vi "helper--Tag Editor.vi"() -> ()   [LabVIEW 2021]
doc: "set the control tags correctly for all of the button types in the directory\n\n<b>Code Developed By:</b>\nTechnology Service Corporation\n1983 S Liberty Drive\nBloomington, IN 47403\nPhone: 812 558-7100\nwww.tsc.com/atcs\n\nDeveloper:\nDaniel Coons"
panel:
  in  "write":bool
  out "Table Control":string[][](table)
  in  "Control":u16(ring) items=["elevated--rectangular--icon.ctl", "elevated--rounded--icon.ctl", "filled--rectangular--icon.ctl", "filled--rounded--icon.ctl", "nooutline--rectangular--icon.ctl", "nooutline--rounded--icon.ctl", "outline--rectangular--icon.ctl", "outline--rounded--icon.ctl", "tonal--rectangular--icon.ctl", "tonal--rounded--icon.ctl", "transparent--rectangular--icon.ctl", "transparent--rounded--icon.ctl", "FAB--icon--rounded.ctl", "nooutline--icon--rectangular--40x40.ctl", "filled--icon--mulitple--rectangular.ctl", "filled--text--rectangular.ctl", "filled--text--rounded.ctl", "nooutline--text--rectangular.ctl", "nooutline--text--rounded.ctl", "outline--text--rectangular.ctl", "outline--text--rounded.ctl", "tonal--text--rectangular.ctl", "tonal--text--rounded.ctl", "token--dark.ctl", "token--light.ctl"]
  in  "Tag Choice":string(combo)
  in  "Tag Value":string="button-type"
  out "error out":errorcluster
  # "legacy categories"
  # "control-level:\nN/A\nPrimary\nSecondary\nTertiary\nError\nPrimary Fixed\nSecondary Fixed\nTertiary Fixed"
  # "boolean-level:\nDefault\nN/A\nNo Change\nNo-Change\nNoChange\nNA"
  # "button-type:\nOutline\nNo-Outline\nTonal\nFilled\nTransparent\nFAB\nElevated"
  # "Control Types:\noutline--icon--rounded\noutline--text--rounded\nnooutline--icon--rounded\nnooutline--text--rounded\ntonal--icon--rounded\ntonal--text--rounded\nfilled--icon--rounded\nfilled--text--rounded"
  # "Control Types:\noutline--icon--rectangular\noutline--text--rectangular\nnooutline--icon--rectangular\nnooutline--text--rectangular\ntonal--icon--rectangular\ntonal--text--rectangular\nfilled--icon--rectangular\nfilled--text--rectangular"
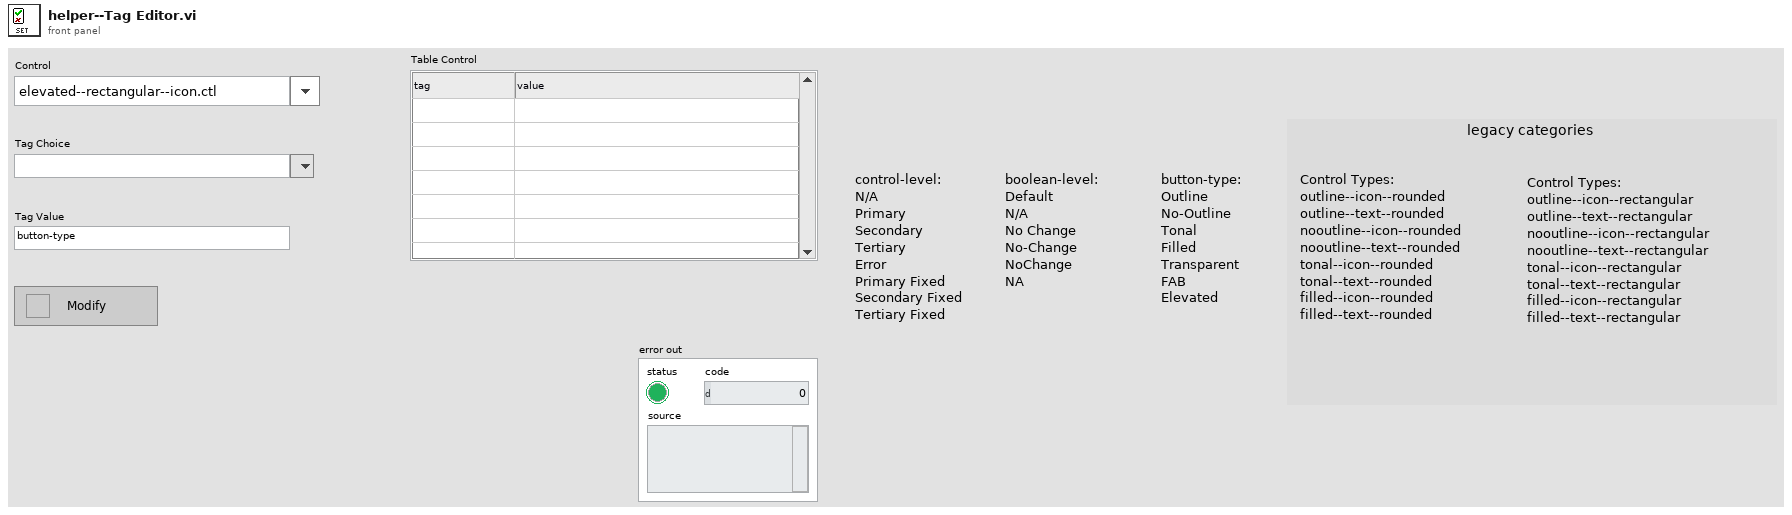
[diagram p1: front panel]
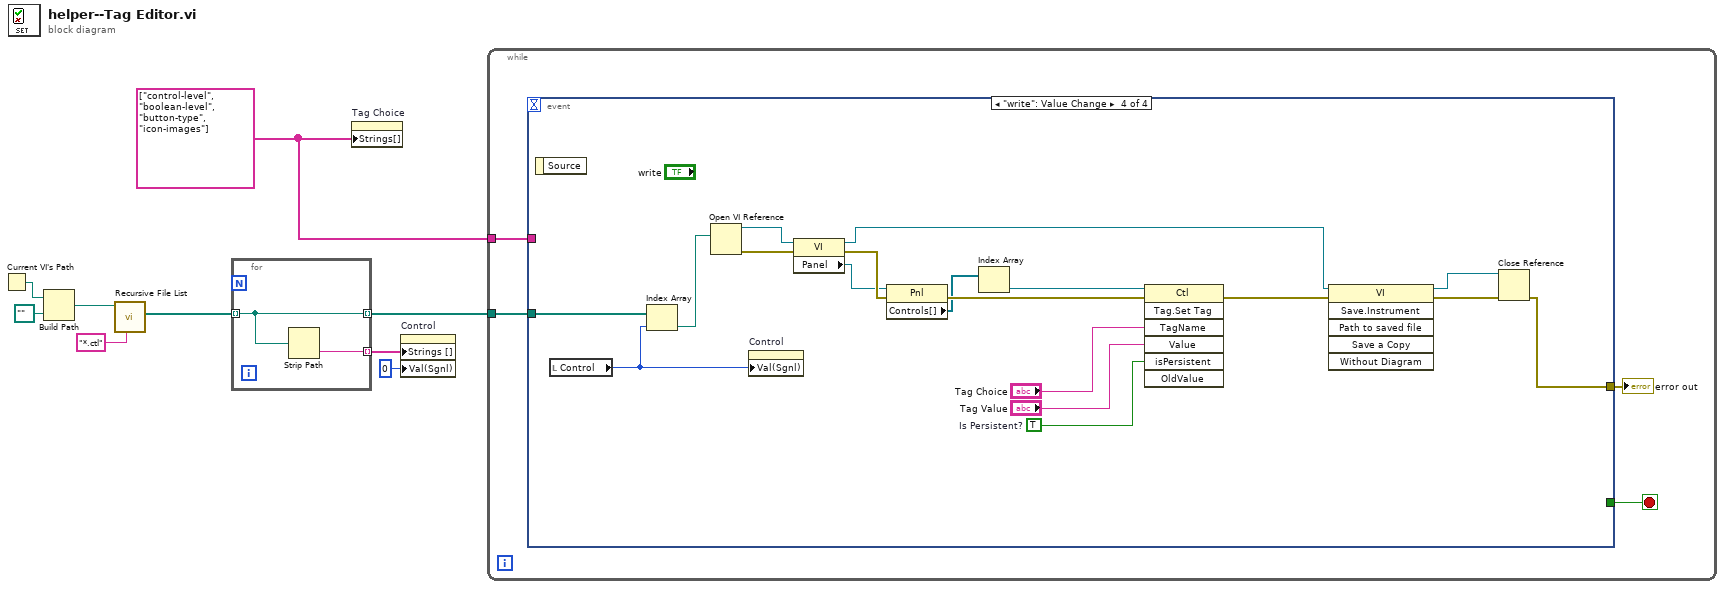
[diagram p0: block diagram]
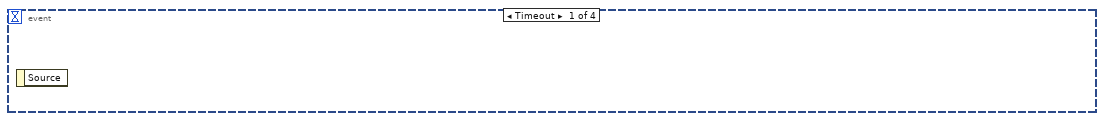
[diagram p2: hidden frame]
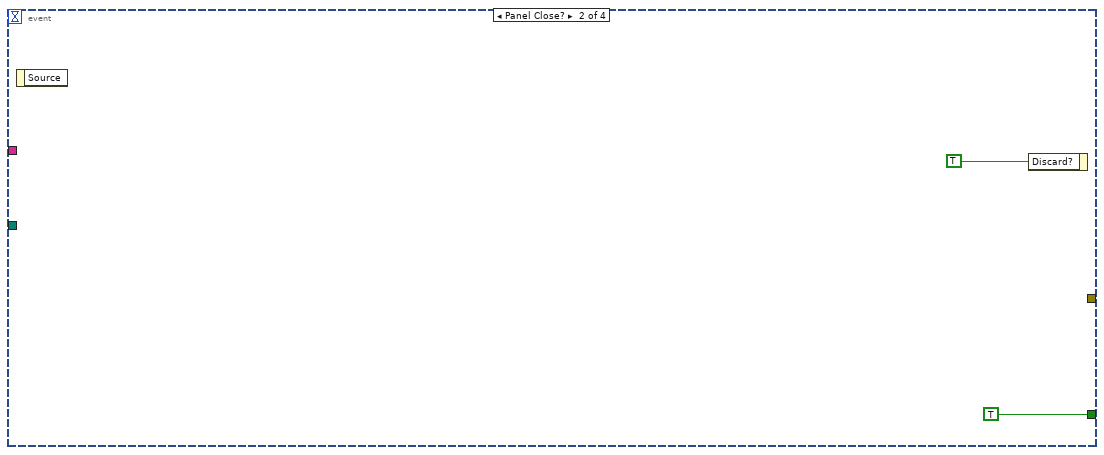
[diagram p3: hidden frame]
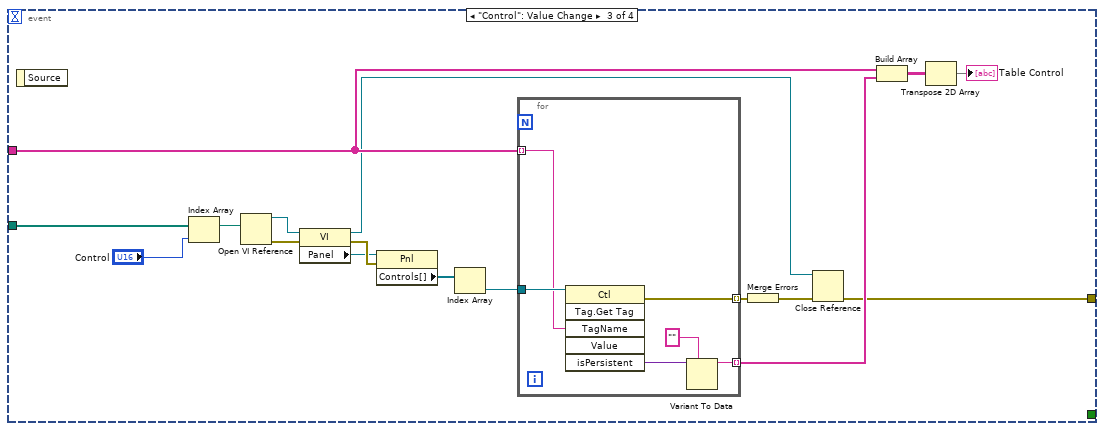
[diagram p4: hidden frame]
diagram:
  w2 = string[] ["control-level", "boolean-level", "button-type", "icon-images"] ("Strings []")
  n1 = Current VI's Path() -> (path=w9:path)
  n2 = Build Path(base path=w9, name or relative path=path "..") -> (appended path=w7:path)
  n3 = call <vilib>:"Recursive File List.vi"("pattern"="*.ctl", "Folder Path"=w7) -> ("All Files in Dir"=w5:path[])  [unwired: 5 in, 4 out]
  n4 = for {
    tunnel: w5 -> [w11] mode=indexing
    tunnel: [w11] -> w4 mode=indexing
    tunnel: [w10] -> w3 mode=indexing
    n5 = Strip Path(path=w11) -> (name=w10:string)  [unwired: 1 out]
  }
  n6 = property on="Tag Choice" class="CmbBox"("Strings[]"=w2) -> ()  [unwired: 2 in, 2 out]
  n7 = property on="Control" class="Ring (strict)"("Strings []"=w3, "Val(Sgnl)"=u16 0 ("Value (Signaling)")) -> ()  [unwired: 2 in, 2 out]
  n8 = while {
    tunnel: w4 -> [w15]
    tunnel: w2 -> [w13]
    stop <- w14 stop-if-true
    n9 = event shown="[3] \"write\": Value Change" {
      selector: _ -> [_ _ _ _]
      dyn-events: _ -> [_ _ _ _]
      timeout: _ -> [_ _ _ _]
      tunnel: [_ _ w18 w41] -> w12
      tunnel: w15 -> [_ _ w28 w45]
      tunnel: [_ TRUE _ _] -> w14
      tunnel: w13 -> [_ _ w24 _]
      event Timeout {
        n10 = event-data() -> ()  [unwired: 1 in, 1 out]
      }
      event Panel Close? {
        n11 = event-data() -> ()  [unwired: 1 in, 1 out]
        n12 = event-data("Discard?"=TRUE) -> ()  [unwired: 1 in, 1 out]
      }
      event "Control": Value Change {
        n13 = event-data() -> ()  [unwired: 1 in, 1 out]
        n14 = Index Array(array=w28, index="Control") -> (element=w29:path)
        n15 = Open VI Reference(vi path=w29) -> (vi reference=w32:refnum<vi>, error out=w34:errorcluster)  [unwired: 5 in]
        n16 = property class="VI"(reference=w32, error in=w34) -> (reference out=w21:refnum<vi>, error out=w33:errorcluster, "Panel"=w31:refnum<vi>)
        n17 = property class="Pnl"(reference=w31, error in=w33) -> ("Controls[]"=w30:refnum<vi>[])  [unwired: 2 out]
        n18 = Index Array(array=w30) -> (element=w26:refnum<vi>)  [unwired: 1 in]
        n19 = for {
          tunnel: w24 -> [w36] mode=indexing
          tunnel: w26 -> [w40]
          tunnel: [w37] -> w23 mode=indexing
          tunnel: [w35] -> w20 mode=indexing
          n20 = invoke class="Ctl" method="Tag.Get Tag"(reference=w40, "TagName"=w36) -> (error out=w35:errorcluster, "isPersistent"=w39:variant)  [unwired: 4 in, 4 out]
          n21 = Variant To Data(type="", Variant=w39) -> (data=w37:string)  [unwired: 1 in, 1 out]
        }
        n22 = Merge Errors(w20) -> (w19:errorcluster)
        n23 = Close Reference(reference=w21, error in (no error)=w19) -> (error out=w18:errorcluster)
        n24 = Build Array(w24, w23) -> (w25:string[][])
        n25 = Transpose 2D Array(2D array=w25) -> (transposed array=→"Table Control":string[][])
      }
      event "write": Value Change {
        w46 = TRUE  # Is Persistent?
        n26 = event-data() -> ()  [unwired: 1 in, 1 out]
        n27 = local read "Control"() -> (w43:u16)
        n28 = Index Array(array=w45, index=w43) -> (element=w47:path)
        n29 = Open VI Reference(vi path=w47) -> (vi reference=w56:refnum<vi>, error out=w58:errorcluster)  [unwired: 5 in]
        n30 = property on="Control" class="Ring (strict)"("Val(Sgnl)"=w43) -> ()  [unwired: 2 in, 2 out]
        n31 = property class="VI"(reference=w56, error in=w58) -> (reference out=w49:refnum<vi>, error out=w57:errorcluster, "Panel"=w54:refnum<vi>)
        n32 = property class="Pnl"(reference=w54, error in=w57) -> (error out=w55:errorcluster, "Controls[]"=w53:refnum<vi>[])  [unwired: 1 out]
        n33 = Index Array(array=w53) -> (element=w51:refnum<vi>)  [unwired: 1 in]
        n34 = invoke class="Ctl" method="Tag.Set Tag"(reference=w51, error in=w55, "TagName"="Tag Choice", "Value"="Tag Value", "isPersistent"=w46) -> (error out=w52:errorcluster)  [unwired: 2 in, 6 out]
        n35 = invoke class="VI" method="Save.Instrument"(reference=w49, error in=w52) -> (reference out=w48:refnum<vi>, error out=w50:errorcluster)  [unwired: 4 in, 4 out]
        n36 = Close Reference(reference=w48, error in (no error)=w50) -> (error out=w41:errorcluster)
      }
    }
    "error out" <- w12
  }
